vi "Parse PS180 Errors.vi"(1 "error in (no error)":errorcluster, 2 "PS 180 String":string) -> (0 "error out":errorcluster)   [LabVIEW 2021]
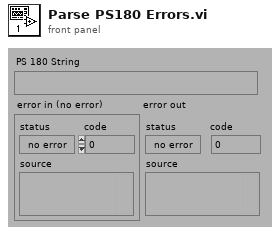
[diagram p1: front panel]
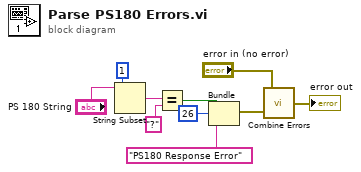
[diagram p0: block diagram]
diagram:
  n1 = String Subset(string="PS 180 String", length (rest)=1) -> (substring=w8:string)  [unwired: 1 in]
  n2 = Equal?(x=w8, y="?") -> (x = y?=w6:bool)
  n3 = Bundle(w6, 26, "PS180 Response Error") -> (w2:errorcluster)  [unwired: 1 in]
  n4 = call "Combine Errors.vi"(1:"error in (no error)"=w2, 2:"error in (no error)"="error in (no error)") -> ("error out"=→"error out":errorcluster)
